vi "Bounds_of_buttons.vi"(11 "Refs cluster In":T2) -> (0 "False Array":bool[](array[boolean]), 2 "Bounds":T1[](array[typedef]), 3 "Refs cluster Out":T2)   [LabVIEW 2015]
uses:
  <vilib>/Utility/miscctls.llb/LVRectTypeDef.ctl
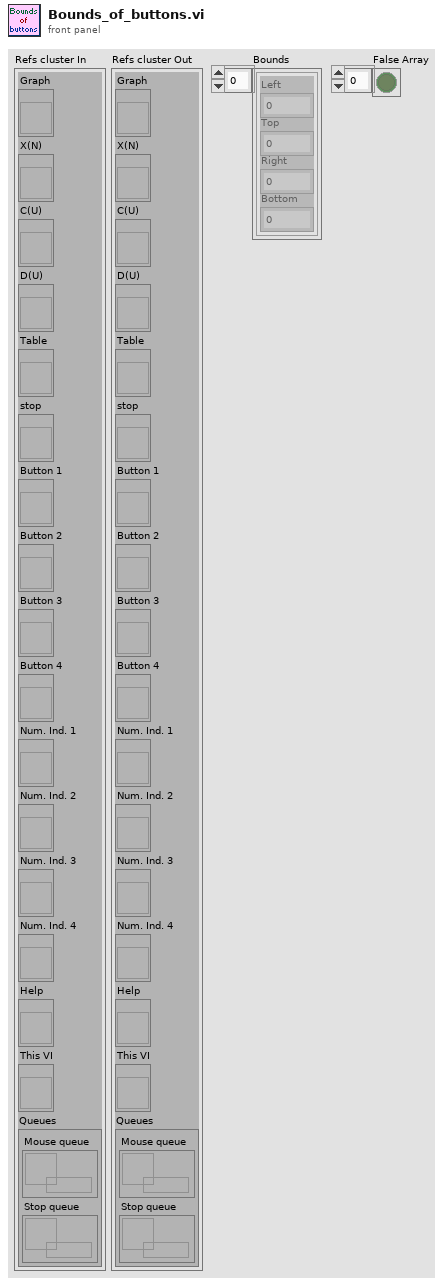
[diagram p1: front panel]
types:
  T1 = typedef "LVRectTypeDef.ctl" = cluster{"Left":i16, "Top":i16, "Right":i16, "Bottom":i16}
  T2 = cluster{"Graph":refnum<vi>, "X(N)":refnum<vi>, "C(U)":refnum<vi>, "D(U)":refnum<vi>, "Table":refnum<vi>, "stop":refnum<vi>, "Button 1":refnum<vi>, "Button 2":refnum<vi>, "Button 3":refnum<vi>, "Button 4":refnum<vi>, "Num. Ind. 1":refnum<vi>, "Num. Ind. 2":refnum<vi>, "Num. Ind. 3":refnum<vi>, "Num. Ind. 4":refnum<vi>, "Help":refnum<vi>, "This VI":refnum<vi>, "Queues":cluster{"Mouse queue":refnum<queue>, "Stop queue":refnum<queue>}}
  T3 = typedef "LVPointTypeDef.ctl" = cluster{"Horizontal":i16, "Vertical":i16}
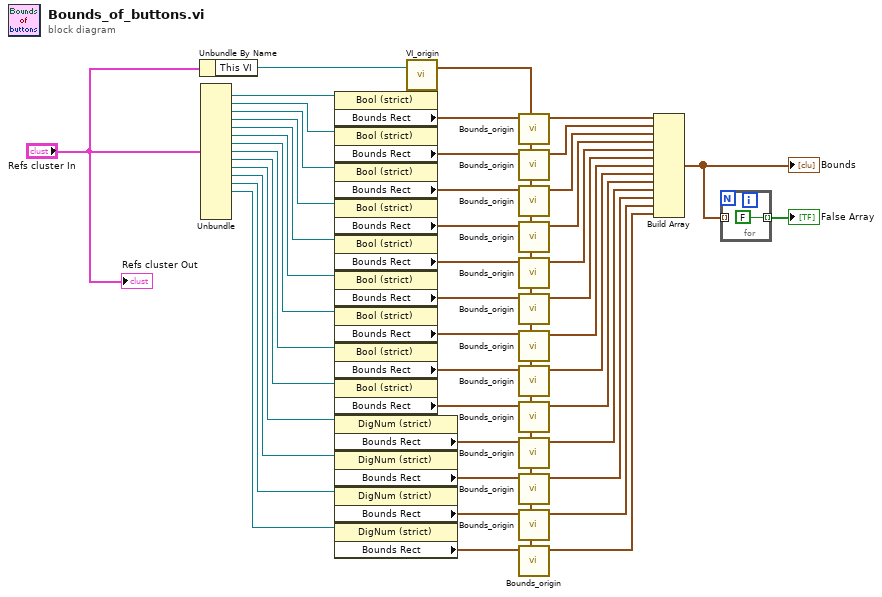
[diagram p0: block diagram]
diagram:
  n1 = Unbundle By Name("Refs cluster In") -> ("This VI"=w2:refnum<vi>)
  n2 = Unbundle("Refs cluster In") -> ("X(N)"=w44:refnum<vi>, "C(U)"=w43:refnum<vi>, "D(U)"=w42:refnum<vi>, "Table"=w41:refnum<vi>, "stop"=w40:refnum<vi>, "Button 1"=w39:refnum<vi>, "Button 2"=w38:refnum<vi>, "Button 3"=w37:refnum<vi>, "Button 4"=w36:refnum<vi>, "Num. Ind. 1"=w35:refnum<vi>, "Num. Ind. 2"=w34:refnum<vi>, "Num. Ind. 3"=w33:refnum<vi>, "Num. Ind. 4"=w32:refnum<vi>)  [unwired: 4 out]
  n3 = property class="Bool (strict)"(reference=w44) -> ("Bounds Rect"=w31:T1)  [unwired: 1 in, 2 out]
  n4 = property class="Bool (strict)"(reference=w43) -> ("Bounds Rect"=w30:T1)  [unwired: 1 in, 2 out]
  n5 = property class="Bool (strict)"(reference=w42) -> ("Bounds Rect"=w29:T1)  [unwired: 1 in, 2 out]
  n6 = property class="Bool (strict)"(reference=w41) -> ("Bounds Rect"=w28:T1)  [unwired: 1 in, 2 out]
  n7 = property class="Bool (strict)"(reference=w40) -> ("Bounds Rect"=w27:T1)  [unwired: 1 in, 2 out]
  n8 = property class="Bool (strict)"(reference=w39) -> ("Bounds Rect"=w26:T1)  [unwired: 1 in, 2 out]
  n9 = property class="Bool (strict)"(reference=w38) -> ("Bounds Rect"=w25:T1)  [unwired: 1 in, 2 out]
  n10 = property class="Bool (strict)"(reference=w37) -> ("Bounds Rect"=w24:T1)  [unwired: 1 in, 2 out]
  n11 = property class="Bool (strict)"(reference=w36) -> ("Bounds Rect"=w23:T1)  [unwired: 1 in, 2 out]
  n12 = property class="DigNum (strict)"(reference=w35) -> ("Bounds Rect"=w22:T1)  [unwired: 1 in, 2 out]
  n13 = property class="DigNum (strict)"(reference=w34) -> ("Bounds Rect"=w21:T1)  [unwired: 1 in, 2 out]
  n14 = property class="DigNum (strict)"(reference=w33) -> ("Bounds Rect"=w20:T1)  [unwired: 1 in, 2 out]
  n15 = property class="DigNum (strict)"(reference=w32) -> ("Bounds Rect"=w19:T1)  [unwired: 1 in, 2 out]
  n16 = call "VI_origin.vi"("VI"=w2) -> ("Origin"=w18:T3)  [unwired: 2 in]
  n17 = call "Bounds_origin.vi"("Origin"=w18, "Bounds In"=w31) -> ("Bounds out"=w17:T1)  [unwired: 9 in]
  n18 = call "Bounds_origin.vi"("Origin"=w18, "Bounds In"=w30) -> ("Bounds out"=w16:T1)  [unwired: 9 in]
  n19 = call "Bounds_origin.vi"("Origin"=w18, "Bounds In"=w29) -> ("Bounds out"=w15:T1)  [unwired: 9 in]
  n20 = call "Bounds_origin.vi"("Origin"=w18, "Bounds In"=w28) -> ("Bounds out"=w14:T1)  [unwired: 9 in]
  n21 = call "Bounds_origin.vi"("Origin"=w18, "Bounds In"=w27) -> ("Bounds out"=w13:T1)  [unwired: 9 in]
  n22 = call "Bounds_origin.vi"("Origin"=w18, "Bounds In"=w26) -> ("Bounds out"=w12:T1)  [unwired: 9 in]
  n23 = call "Bounds_origin.vi"("Origin"=w18, "Bounds In"=w25) -> ("Bounds out"=w11:T1)  [unwired: 9 in]
  n24 = call "Bounds_origin.vi"("Origin"=w18, "Bounds In"=w24) -> ("Bounds out"=w10:T1)  [unwired: 9 in]
  n25 = call "Bounds_origin.vi"("Origin"=w18, "Bounds In"=w23) -> ("Bounds out"=w9:T1)  [unwired: 9 in]
  n26 = call "Bounds_origin.vi"("Origin"=w18, "Bounds In"=w22) -> ("Bounds out"=w8:T1)  [unwired: 9 in]
  n27 = call "Bounds_origin.vi"("Origin"=w18, "Bounds In"=w21) -> ("Bounds out"=w7:T1)  [unwired: 9 in]
  n28 = call "Bounds_origin.vi"("Origin"=w18, "Bounds In"=w20) -> ("Bounds out"=w6:T1)  [unwired: 9 in]
  n29 = call "Bounds_origin.vi"("Origin"=w18, "Bounds In"=w19) -> ("Bounds out"=w5:T1)  [unwired: 9 in]
  n30 = Build Array(w17, w16, w15, w14, w13, w12, w11, w10, w9, w8, w7, w6, w5) -> (w4:T1[])
  "Bounds" <- w4
  n31 = for {
    tunnel: [FALSE] -> w1 mode=indexing
    tunnel: w4 -> [_] mode=indexing
  }
  "False Array" <- w1
  "Refs cluster Out" <- "Refs cluster In"
